vi "textColor.vi"(8 "Error In":errorcluster, 11 "QTextEdit In":refnum<class "QTextEdit.lvclass">) -> (0 "Error Out":errorcluster, 2 "Value":refnum<class "QColor.lvclass">, 3 "QTextEdit Out":refnum<class "QTextEdit.lvclass">)   [LabVIEW 2014, in "QTextEdit.lvclass"]
doc: "LabVIEW-specific documentation is not yet available. See <b>http://doc.qt.io/qt-5/QTextEdit.html#textColor</b>"
uses:
  QTextEdit.lvclass
  Qt GUI/QColor/QColor.lvclass
  LQ Core/LQIdentity/LQIdentity.lvclass/LQIdentity.ctl
  LQ Core/LQSerialData/LQSerialData.lvclass/LQSerialData.ctl
  LQ Core/LQ Core.lvlib
  LQ Core/LQIdentity/LQIdentity.lvclass
  LQ Core/LQSerialData/LQSerialData.lvclass
panel:
  # "Copyright (c) 2016 Sze Howe Koh\n\nThis Source Code Form is subject to the terms of the Mozilla Public\nLicense, v. 2.0. If a copy of the MPL was not distributed with this\nfile, You can obtain one at http://mozilla.org/MPL/2.0/."
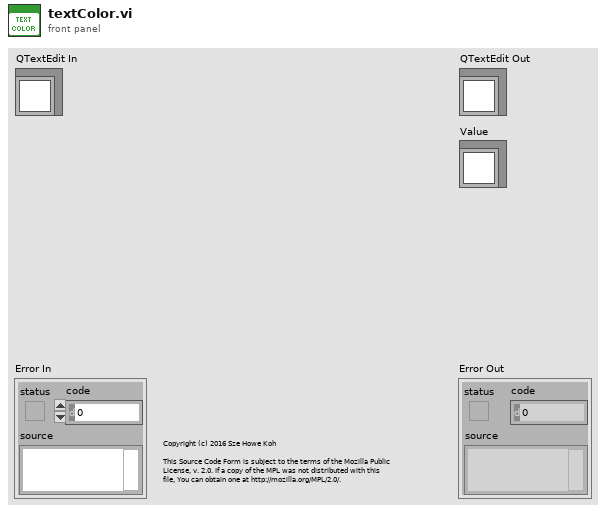
[diagram p1: front panel]
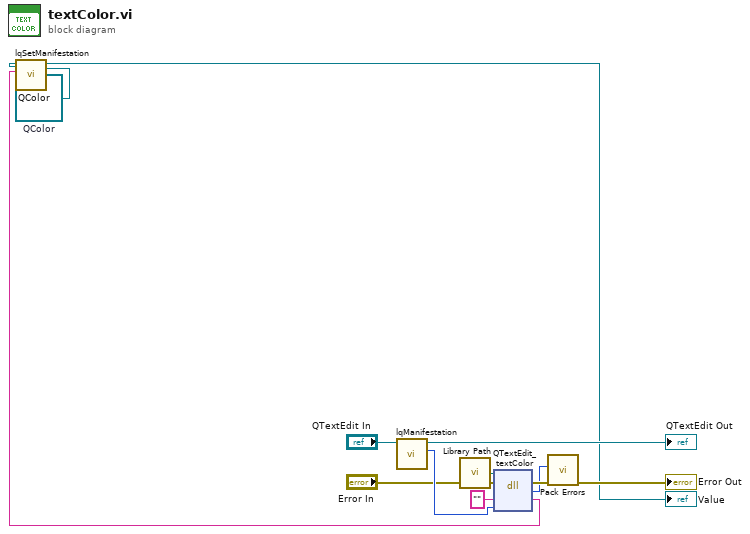
[diagram p0: block diagram]
diagram:
  w1 = refnum<class "QColor.lvclass"> refnum  # QColor
  n1 = call "lqManifestation.vi"("LQIdentity in"="QTextEdit In") -> ("Manifestation"=w8:u64, "LQIdentity out"=→"QTextEdit Out":refnum<class "QTextEdit.lvclass">)  [unwired: 9 in]
  n2 = call "Library Path.vi"() -> ("Library Path"=w9:path)
  n3 = dll-call lib="?" fn="QTextEdit_textColor"(path in=w9, error in="Error In", "_retVal"="" ("retVal"), "_instance"=w8) -> (error out=w6:errorcluster, w4:i32, "_retVal"=w2:string)  [unwired: 2 in, 1 out]
  n4 = call "lqSetManifestation.vi"("Manifestation"=w2, "LQSerialData in"=w1) -> ("LQSerialData out"=→"Value":refnum<class "QColor.lvclass">)  [unwired: 8 in, 1 out]
  n5 = call "Pack Errors.vi"("Error In"=w6, "Error Code"=w4) -> ("Error Out"=→"Error Out":errorcluster)  [unwired: 9 in]
